vi "超标浓度设置.vi"() -> ()   [LabVIEW 2016, in "超标留样集成.lvlib"]
uses:
  <vilib>/Utility/miscctls.llb/LVPointTypeDef.ctl
  <vilib>/Utility/config.llb/NI_LVConfig.lvlib
panel:
  in  "PH下限浓度":dbl
  in  "取消":bool
  in  "确定":bool
  in  "氨氮超标浓度":dbl
  in  "总磷超标浓度":dbl
  in  "总氮超标浓度":dbl
  in  "CODMn超标浓度":dbl
  in  "CODCr超标浓度":dbl
  in  "PH超标浓度":dbl
  in  "溶解氧下限浓度":dbl
  in  "电导率超标浓度":dbl
  in  "浊度超标浓度":dbl
  in  "叶绿素a超标浓度":dbl
  in  "藻密度超标浓度":dbl
  in  "蓝绿藻超标浓度":dbl
  in  "ORP超标浓度":dbl
  in  "COD超标浓度":dbl
  in  "铅超标浓度":dbl
  in  "镉超标浓度":dbl
  in  "铜超标浓度":dbl
  in  "锌超标浓度":dbl
  in  "镍超标浓度":dbl
  in  "锰超标浓度":dbl
  in  "汞超标浓度":dbl
  # "超标浓度报警配置"
  # "cells/mL"
  # "mg/L"
  # "/"
  # "cells/mL"
  # "/"
  # "mg/L"
  # "mg/L"
  # "/"
  # "mg/L"
  # "μs/cm"
  # "mg/L"
  # "mg/L"
  # "NTU"
  # "mg/L"
  # "μg/L"
  # "mg/L"
  # "mg/L"
  # "mg/L"
  # "mg/L"
  # "mg/L"
  # "mg/L"
  # "mg/L"
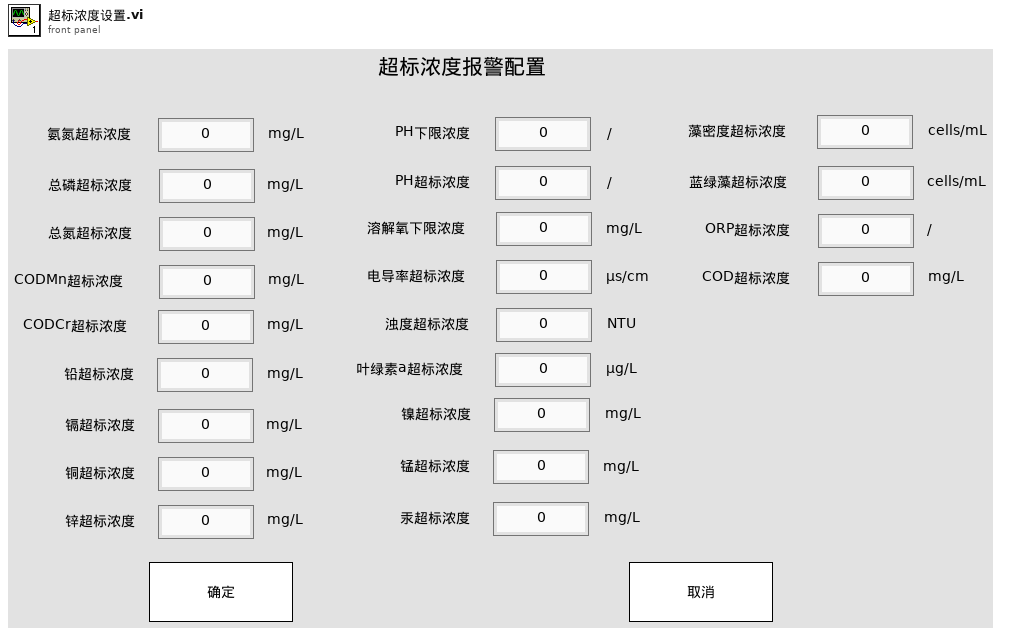
[diagram p1: front panel]
types:
  T1 = typedef "LVPointTypeDef.ctl" = cluster{"Horizontal":i16, "Vertical":i16}
  T2 = typedef "NI_LVConfig.lvlib/Config Data RefNum.ctl" = refnum<k1>
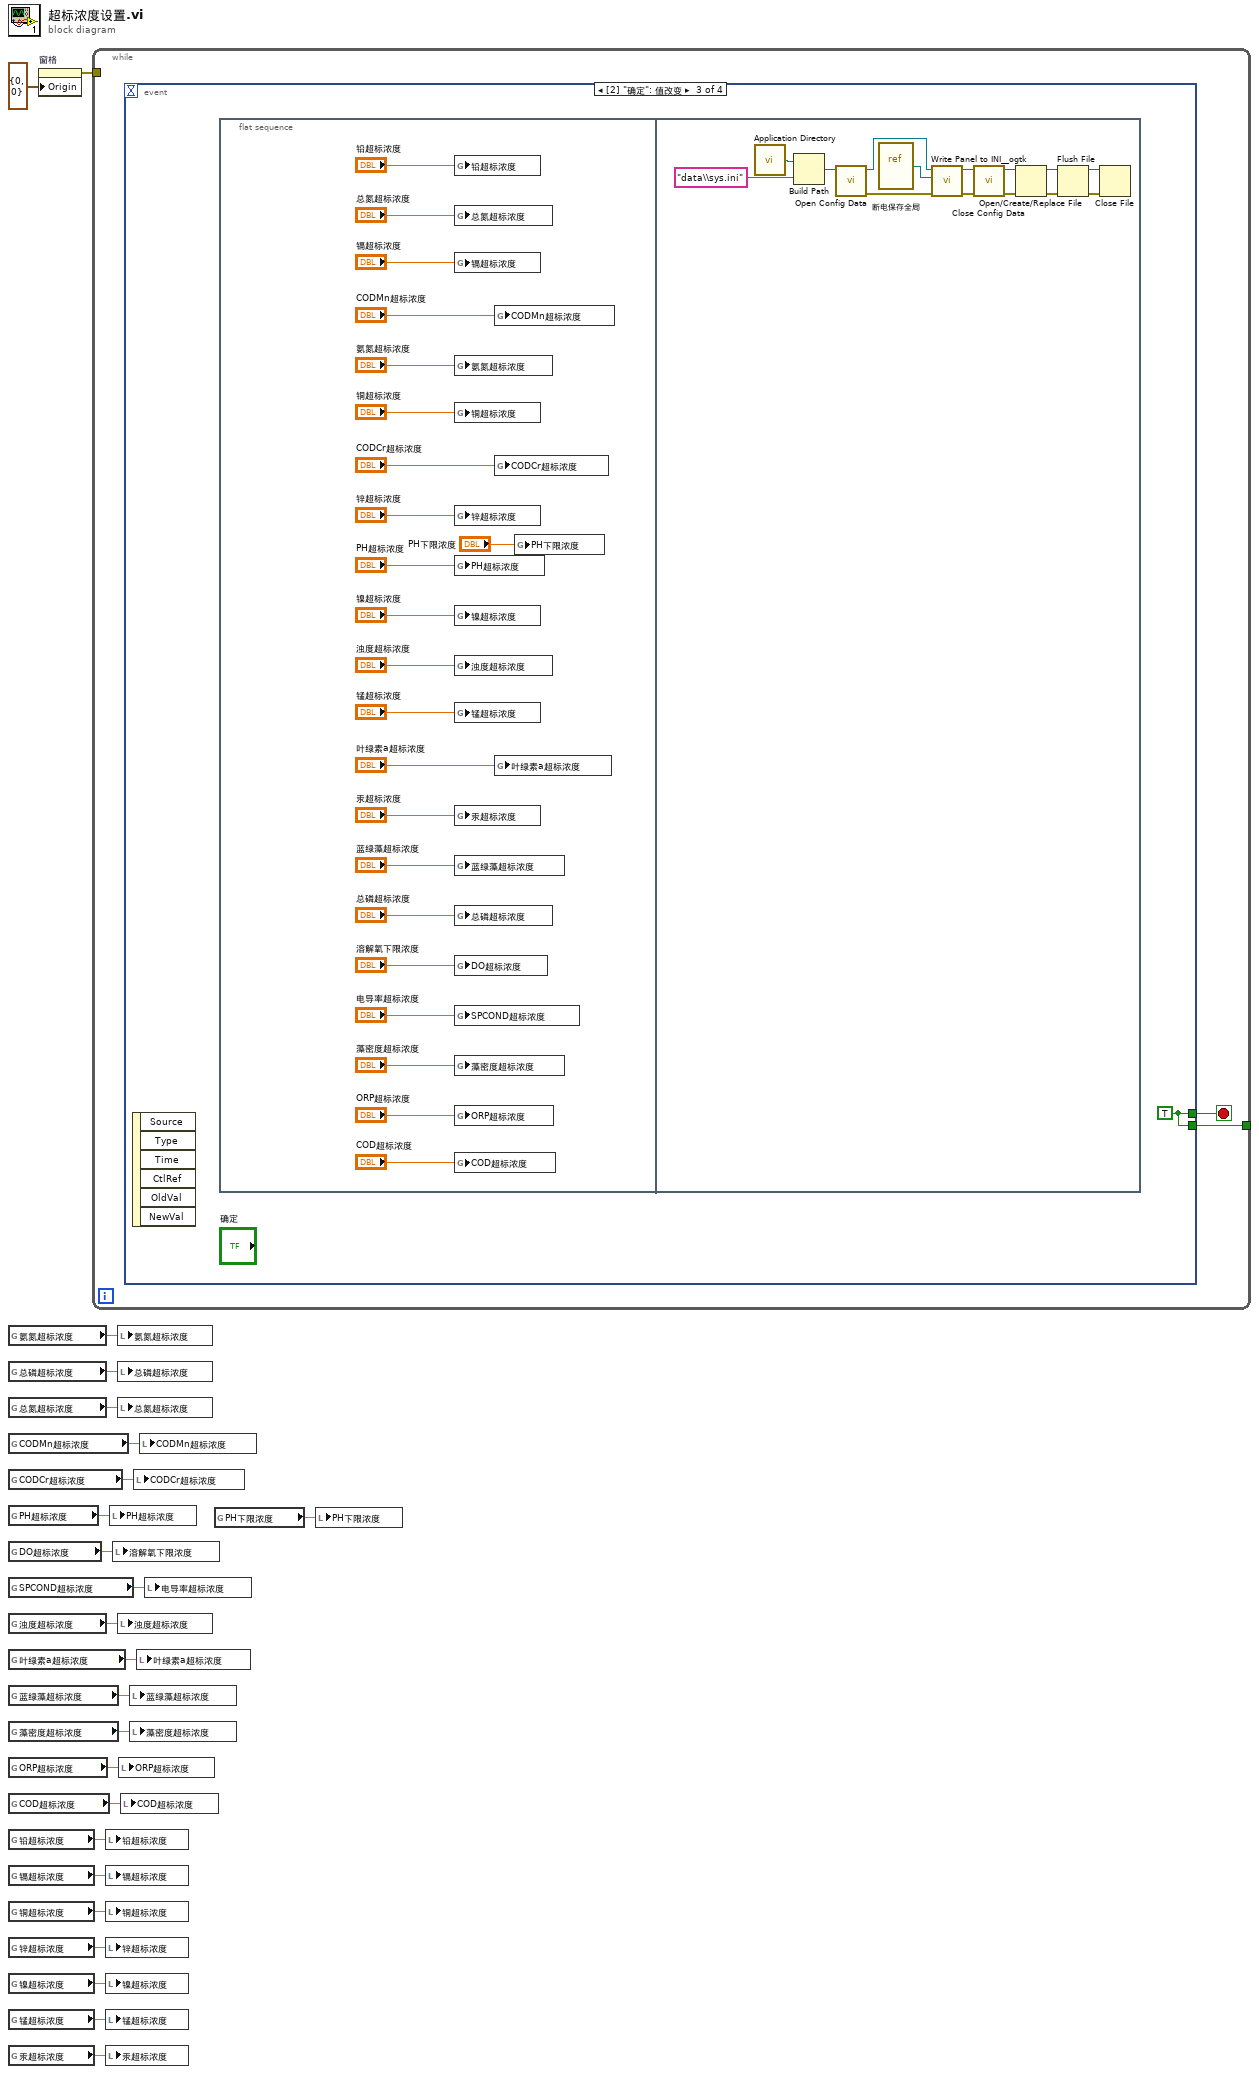
[diagram p0: block diagram]
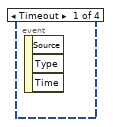
[diagram p2: hidden frame]
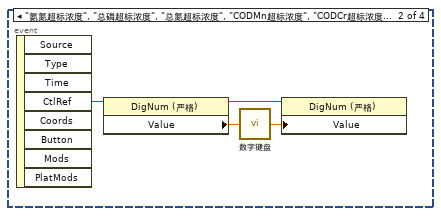
[diagram p3: hidden frame]
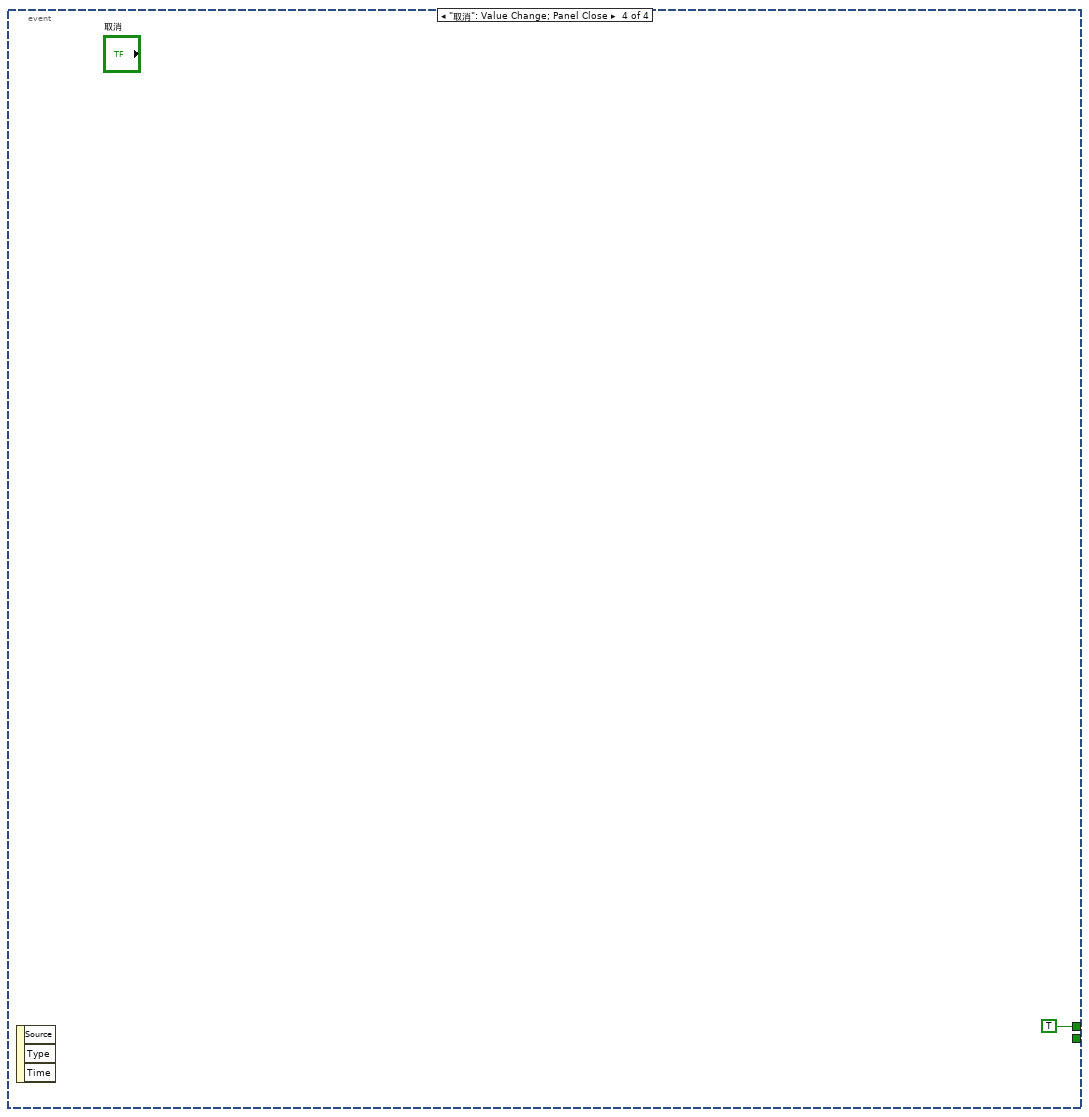
[diagram p4: hidden frame]
diagram:
  n1 = global read "断电保存全局.vi" "氨氮超标浓度"() -> (w22:dbl)
  n2 = global read "断电保存全局.vi" "总磷超标浓度"() -> (w21:dbl)
  n3 = global read "断电保存全局.vi" "总氮超标浓度"() -> (w20:dbl)
  n4 = global read "断电保存全局.vi" "CODMn超标浓度"() -> (w19:dbl)
  n5 = global read "断电保存全局.vi" "CODCr超标浓度"() -> (w18:dbl)
  n6 = global read "断电保存全局.vi" "PH超标浓度"() -> (w17:dbl)
  n7 = global read "断电保存全局.vi" "DO超标浓度"() -> (w16:dbl)
  n8 = global read "断电保存全局.vi" "SPCOND超标浓度"() -> (w15:dbl)
  n9 = global read "断电保存全局.vi" "浊度超标浓度"() -> (w14:dbl)
  n10 = global read "断电保存全局.vi" "叶绿素a超标浓度"() -> (w13:dbl)
  n11 = global read "断电保存全局.vi" "蓝绿藻超标浓度"() -> (w12:dbl)
  n12 = global read "断电保存全局.vi" "藻密度超标浓度"() -> (w11:dbl)
  n13 = global read "断电保存全局.vi" "ORP超标浓度"() -> (w10:dbl)
  n14 = global read "断电保存全局.vi" "COD超标浓度"() -> (w9:dbl)
  n15 = global read "断电保存全局.vi" "铅超标浓度"() -> (w8:dbl)
  n16 = global read "断电保存全局.vi" "镉超标浓度"() -> (w7:dbl)
  n17 = global read "断电保存全局.vi" "铜超标浓度"() -> (w6:dbl)
  n18 = global read "断电保存全局.vi" "锌超标浓度"() -> (w5:dbl)
  n19 = global read "断电保存全局.vi" "镍超标浓度"() -> (w4:dbl)
  n20 = global read "断电保存全局.vi" "锰超标浓度"() -> (w3:dbl)
  n21 = global read "断电保存全局.vi" "汞超标浓度"() -> (w2:dbl)
  n22 = property on="窗格" class="Pane"("Origin"=T1 {"Horizontal"=0, "Vertical"=0} ("原点")) -> (error out=w23:errorcluster)  [unwired: 2 in, 1 out]
  n23 = while {
    tunnel: [w25] -> _
    tunnel: w23 -> [_]
    stop <- w26 stop-if-true
    n24 = event shown="[2] \"确定\": 值改变" {
      selector: _ -> [_ _ _ _]
      dyn-events: _ -> [_ _ _ _]
      timeout: _ -> [_ _ _ _]
      tunnel: [_ _ w31 TRUE] -> w26
      tunnel: [_ _ w31 _] -> w25
      event Timeout {
        n25 = event-data() -> ()  [unwired: 1 in, 3 out]
      }
      event "氨氮超标浓度", "总磷超标浓度", "总氮超标浓度", "CODMn超标浓度", "CODCr超标浓度", "PH超标浓度", "溶解氧下限浓度", "电导率超标浓度", "浊度超标浓度", "叶绿素a超标浓度", "藻密度超标浓度", "蓝绿藻超标浓度", "ORP超标浓度", "COD超标浓度", "铅超标浓度", "镉超标浓度", "铜超标浓度", "锌超标浓度", "镍超标浓度", "锰超标浓度", "汞超标浓度", "PH下限浓度": Mouse Down {
        n26 = event-data() -> ("CtlRef"=w30:refnum<vi>)  [unwired: 1 in, 7 out]
        n27 = property class="DigNum (严格)"(reference=w30) -> (reference out=w28:refnum<vi>, "Value"=w29:dbl)  [unwired: 1 in, 1 out]
        n28 = call "数字键盘.vi"("OldNumber"=w29) -> ("NewNumber"=w27:sgl)
        n29 = property class="DigNum (严格)"(reference=w28, "Value"=w27) -> ()  [unwired: 1 in, 2 out]
      }
      event "确定": Value Change {
        w31 = TRUE
        n30 = event-data() -> ()  [unwired: 1 in, 6 out]
        n31 = flat-sequence {
          frame #0 {
            n32 = global write "断电保存全局.vi" "铅超标浓度"("铅超标浓度") -> ()
            n33 = global write "断电保存全局.vi" "总氮超标浓度"("总氮超标浓度") -> ()
            n34 = global write "断电保存全局.vi" "镉超标浓度"("镉超标浓度") -> ()
            n35 = global write "断电保存全局.vi" "氨氮超标浓度"("氨氮超标浓度") -> ()
            n36 = global write "断电保存全局.vi" "铜超标浓度"("铜超标浓度") -> ()
            n37 = global write "断电保存全局.vi" "锌超标浓度"("锌超标浓度") -> ()
            n38 = global write "断电保存全局.vi" "PH超标浓度"("PH超标浓度") -> ()
            n39 = global write "断电保存全局.vi" "镍超标浓度"("镍超标浓度") -> ()
            n40 = global write "断电保存全局.vi" "浊度超标浓度"("浊度超标浓度") -> ()
            n41 = global write "断电保存全局.vi" "锰超标浓度"("锰超标浓度") -> ()
            n42 = global write "断电保存全局.vi" "汞超标浓度"("汞超标浓度") -> ()
            n43 = global write "断电保存全局.vi" "蓝绿藻超标浓度"("蓝绿藻超标浓度") -> ()
            n44 = global write "断电保存全局.vi" "总磷超标浓度"("总磷超标浓度") -> ()
            n45 = global write "断电保存全局.vi" "DO超标浓度"("溶解氧下限浓度") -> ()
            n46 = global write "断电保存全局.vi" "SPCOND超标浓度"("电导率超标浓度") -> ()
            n47 = global write "断电保存全局.vi" "藻密度超标浓度"("藻密度超标浓度") -> ()
            n48 = global write "断电保存全局.vi" "ORP超标浓度"("ORP超标浓度") -> ()
            n49 = global write "断电保存全局.vi" "COD超标浓度"("COD超标浓度") -> ()
            n50 = global write "断电保存全局.vi" "CODMn超标浓度"("CODMn超标浓度") -> ()
            n51 = global write "断电保存全局.vi" "CODCr超标浓度"("CODCr超标浓度") -> ()
            n52 = global write "断电保存全局.vi" "叶绿素a超标浓度"("叶绿素a超标浓度") -> ()
            n53 = global write "断电保存全局.vi" "PH下限浓度"("PH下限浓度") -> ()
          }
          frame #1 {
            n54 = call <vilib>:"Application Directory.vi"() -> ("Application Directory"=w55:path)
            n55 = Build Path(base path=w55, name or relative path="data\\sys.ini" ("名称或相对路径")) -> (appended path=w56:path)
            n56 = call <vilib>:"Open Config Data.vi"("configuration file path"=w56) -> ("error out"=w60:errorcluster, "refnum"=w57:T2)  [unwired: 8 in, 1 out]
            n57 = vi-ref "断电保存全局.vi"() -> (w58:refnum<vi>)
            n58 = call <userlib>:"Write Panel to INI__ogtk.vi"("error in (no error)"=w60, "VI ref"=w58, "refnum"=w57) -> ("error out"=w61:errorcluster, "refnum out"=w59:T2)  [unwired: 7 in]
            n59 = call <vilib>:"Close Config Data.vi"("error in (no error)"=w61, "refnum"=w59) -> ("error out"=w66:errorcluster, "file path"=w67:path)  [unwired: 8 in]
            n60 = Open/Create/Replace File(file path (use dialog)=w67, error in=w66) -> (refnum out=w63:refnum<file>, error out=w62:errorcluster)  [unwired: 4 in, 1 out]
            n61 = Flush File(refnum=w63, error in=w62) -> (refnum out=w64:refnum<file>, error out=w65:errorcluster)
            n62 = Close File(refnum=w64, error in=w65) -> ()  [unwired: 2 out]
          }
        }
      }
      event "取消": Value Change; Panel Close {
        n63 = event-data() -> ()  [unwired: 1 in, 3 out]
      }
    }
  }
  n64 = local write "铅超标浓度"(w8) -> ()
  n65 = local write "镉超标浓度"(w7) -> ()
  n66 = local write "铜超标浓度"(w6) -> ()
  n67 = local write "锌超标浓度"(w5) -> ()
  n68 = local write "镍超标浓度"(w4) -> ()
  n69 = local write "锰超标浓度"(w3) -> ()
  n70 = local write "汞超标浓度"(w2) -> ()
  n71 = local write "PH超标浓度"(w17) -> ()
  n72 = local write "溶解氧下限浓度"(w16) -> ()
  n73 = local write "氨氮超标浓度"(w22) -> ()
  n74 = local write "总磷超标浓度"(w21) -> ()
  n75 = local write "总氮超标浓度"(w20) -> ()
  n76 = local write "浊度超标浓度"(w14) -> ()
  n77 = local write "ORP超标浓度"(w10) -> ()
  n78 = local write "COD超标浓度"(w9) -> ()
  n79 = local write "蓝绿藻超标浓度"(w12) -> ()
  n80 = local write "藻密度超标浓度"(w11) -> ()
  n81 = local write "CODCr超标浓度"(w18) -> ()
  n82 = local write "叶绿素a超标浓度"(w13) -> ()
  n83 = local write "CODMn超标浓度"(w19) -> ()
  n84 = local write "电导率超标浓度"(w15) -> ()
  n85 = global read "断电保存全局.vi" "PH下限浓度"() -> (w1:dbl)
  n86 = local write "PH下限浓度"(w1) -> ()
